vi "Temperature Monitoring.vi"() -> ()   [LabVIEW 2019]
uses:
  <vilib>/Skyline/Tag/Shared/typedefs/DataType.ctl
  <vilib>/Skyline/Configuration/Configuration HTTP_class/Open Configuration HTTP.vi
  <vilib>/Skyline/Tag/Wrapper/Wrapper HTTP_class/Open Tag HTTP.vi
  <vilib>/Skyline/Tag/Wrapper/Wrapper_class/Write Tag (DBL).vi
  <vilib>/Skyline/Tag/Wrapper/Wrapper_class/Close Tag (Single).vi
  <vilib>/Skyline/Configuration/Configuration HTTP_class/NI Skyline Configuration HTTP.lvclass
  <vilib>/Skyline/Configuration/Configuration_class/NI Skyline Configuration.lvclass
  <vilib>/Skyline/Tag/Wrapper/Wrapper_class/NI Skyline Tag.lvclass
  <vilib>/Skyline/Tag/Shared/NI Skyline Tag.lvlib
  <vilib>/Skyline/Tag/Wrapper/Wrapper HTTP_class/NI Skyline Tag HTTP.lvclass
panel:
  in  "Stop":bool
  out "Temperature History":dbl[][](graph)
  out "Temperatures":dbl[](array[numeric])
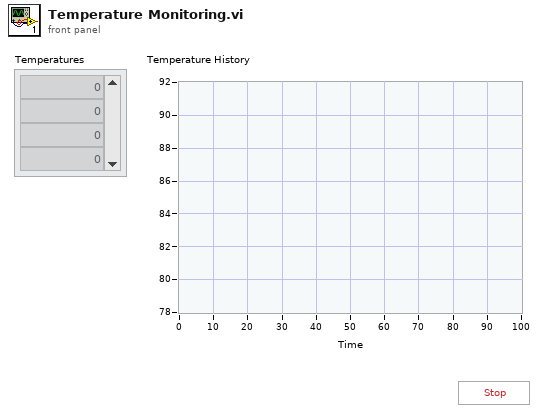
[diagram p1: front panel]
types:
  T1 = typedef "NI Skyline Tag.lvlib/DataType.ctl" = enum32{"Double", "I32", "String", "Boolean", "U64", "Timestamp"}
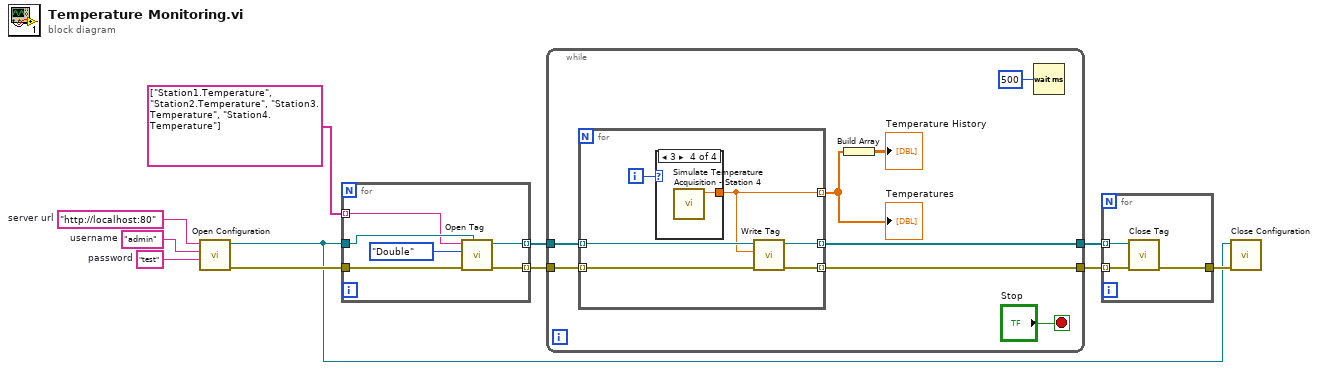
[diagram p0: block diagram]
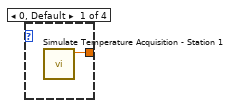
[diagram p2: hidden frame]
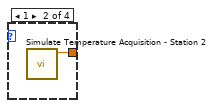
[diagram p3: hidden frame]
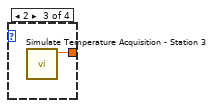
[diagram p4: hidden frame]
diagram:
  w1 = "test"  # password
  w2 = "admin"  # username
  w3 = "http://localhost:80"  # server url
  n1 = call-poly <vilib>:"Open Configuration.vi"("password"=w1, "username"=w2, "server url"=w3) -> ("error out"=w11:errorcluster, "HTTP configuration out"=w4:refnum<class "NI Skyline Configuration HTTP.lvclass">)  [unwired: 7 in]
  n2 = for {
    tunnel: w11 -> [w17]
    tunnel: w4 -> [w16]
    tunnel: string[] ["Station1.Temperature", "Station2.Temperature", "Station3.Temperature", "Station4.Temperature"] -> [w14] mode=indexing
    tunnel: [w13] -> w9 mode=indexing
    tunnel: [w12] -> w8 mode=indexing
    n3 = call-poly <vilib>:"Open Tag.vi"("configuration"=w16, "error in (no error)"=w17, "Data Type"=DataType."Double", "path"=w14) -> ("error out"=w12:errorcluster, "tag out"=w13:refnum<class "NI Skyline Tag.lvclass">)  [unwired: 6 in]
  }
  n4 = while {
    tunnel: w9 -> [w25]
    tunnel: w8 -> [w24]
    tunnel: [w23] -> w7
    tunnel: [w22] -> w6
    stop <- "Stop" stop-if-true
    n5 = for {
      tunnel: w25 -> [w31] mode=indexing
      tunnel: w24 -> [w30] mode=indexing
      tunnel: [w29] -> w22 mode=indexing
      tunnel: [w28] -> w23 mode=indexing
      tunnel: [w26] -> w20 mode=indexing
      i -> [w27]
      n6 = case shown="3" w27 {
        tunnel: [w32 w33 w34 w35] -> w26
        frame 0, Default {
          n7 = call "Simulate Temperature Acquisition - Station 1.vi"() -> ("Temperature"=w32:dbl)  [unwired: 11 in]
        }
        frame 1 {
          n8 = call "Simulate Temperature Acquisition - Station 2.vi"() -> ("Temperature"=w33:dbl)  [unwired: 11 in]
        }
        frame 2 {
          n9 = call "Simulate Temperature Acquisition - Station 3.vi"() -> ("Temperature"=w34:dbl)  [unwired: 11 in]
        }
        frame 3 {
          n10 = call "Simulate Temperature Acquisition - Station 4.vi"() -> ("Temperature"=w35:dbl)  [unwired: 11 in]
        }
      }
      n11 = call-poly <vilib>:"Write Tag.vi"("error in (no error)"=w30, "value"=w26, "tag in"=w31) -> ("error out"=w29:errorcluster, "tag out"=w28:refnum<class "NI Skyline Tag.lvclass">)  [unwired: 7 in]
    }
    "Temperatures" <- w20
    n12 = Build Array(w20) -> (→"Temperature History":dbl[][])
    n13 = Wait (ms)(milliseconds to wait=u32 500) -> ()  [unwired: 1 out]
  }
  n14 = for {
    tunnel: w7 -> [w38] mode=indexing
    tunnel: w6 -> [w37] mode=indexing
    tunnel: [w36] -> w5
    n15 = call-poly <vilib>:"Close Tag.vi"("error in (no error)"=w37, "tag in"=w38) -> ("error out"=w36:errorcluster)  [unwired: 9 in]
  }
  n16 = call-dynamic "Close Configuration.vi"("error in (no error)"=w5, "HTTP configuration in"=w4) -> ()  [unwired: 9 in, 1 out]
